vi "Decompose LabVIEW Object - Child - Private Data Cluster Value.vi"() -> ()   [LabVIEW 2017, in "Composition.Tests.lvlib"]
uses:
  Composition.Tests.lvlib
  Classes/Child/Child.lvclass
  Composition/Composition.lvlib
  <vilib>/addons/_JKI Toolkits/Caraya/classes/Test/Test.lvclass
  <vilib>/addons/_JKI Toolkits/Caraya/classes/Assert/Assert.lvclass
panel:
  out "error out":errorcluster
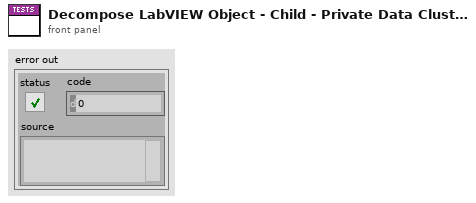
[diagram p1: front panel]
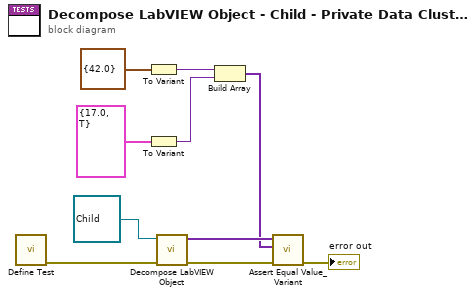
[diagram p0: block diagram]
diagram:
  n1 = call <vilib>:"Define Test.vi"() -> ("error out"=w1:errorcluster)  [unwired: 11 in]
  n2 = To Variant(anything=cluster{"Length":dbl} {"Length"=42.0}) -> (Variant=w5:variant)
  n3 = To Variant(anything=cluster{"Offset":dbl, "Ignored":bool} {"Offset"=17.0, "Ignored"=TRUE}) -> (Variant=w4:variant)
  n4 = call "Decompose LabVIEW Object.vi"("error in (no error)"=w1, "LabVIEW Object"=refnum<class "Child.lvclass"> refnum ("Reflection.Tests.lvlib:Child.lvclass")) -> ("error out"=w9:errorcluster, "Private Data Clusters"=w3:variant[])  [unwired: 6 in, 2 out]
  n5 = Build Array(w5, w4) -> (w2:variant[])
  n6 = call <vilib>:"Assert Equal Value_Variant.vi"("error in (no error)"=w9, "Y"=w2, "X"=w3) -> ("error out"=→"error out":errorcluster)  [unwired: 8 in]
